vi "rethinkdb_msg_split.vi"(8 "error in (no error)":errorcluster, 11 "data in":string) -> (0 "error out":errorcluster, 2 "unterminated?":bool, 3 "messages":string[](array[string]))   [LabVIEW 2017]
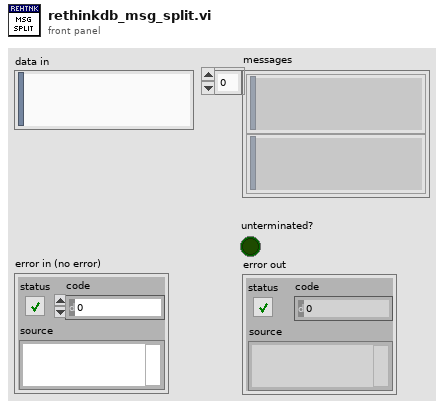
[diagram p1: front panel]
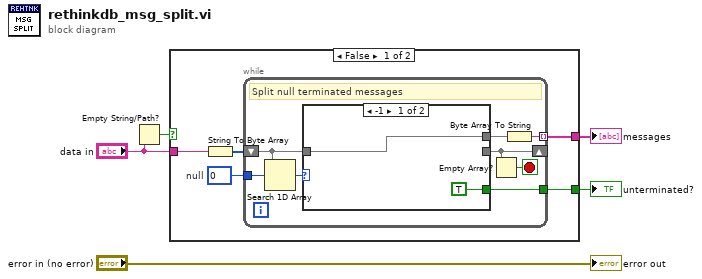
[diagram p0: block diagram]
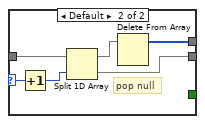
[diagram p2: hidden frame]
diagram:
  n1 = Empty String/Path?(string/path="data in") -> (empty?=w2:bool)
  n2 = case shown="False" w2 {
    tunnel: "data in" -> [w9 _]
    tunnel: [w7 _] -> w5
    tunnel: [w6 _] -> w1
    frame False {
      w10 = u8 0  # null
      n3 = String To Byte Array(string=w9) -> (unsigned byte array=w8:u8[])
      n4 = while {
        tunnel: w10 -> [w18]
        shift-right: [w13] -> _
        shift-left: w8 -> [w17]
        tunnel: [w14] -> w7 mode=indexing
        tunnel: [w11] -> w6
        stop <- w12 stop-if-true
        # "Split null terminated messages"
        n5 = Search 1D Array(1D array=w17, element=w18) -> (index of element=w16:i32)  [unwired: 1 in]
        n6 = case shown="-1" w16 {
          selector: w16 -> [_ w25]
          tunnel: w17 -> [w20 w26]
          tunnel: [_ w24] -> w13
          tunnel: [w20 w21] -> w15
          tunnel: [TRUE _] -> w11
          frame -1 {
          }
          frame Default {
            # "pop null"
            n7 = Increment(x=w25) -> (x+1=w23:i32)
            n8 = Split 1D Array(array=w26, index=w23) -> (first subarray=w22:u8[], second subarray=w24:u8[])
            n9 = Delete From Array(array=w22) -> (array with subset deleted=w21:u8[])  [unwired: 2 in, 1 out]
          }
        }
        n10 = Empty Array?(array=w13) -> (empty?=w12:bool)
        n11 = Byte Array To String(unsigned byte array=w15) -> (string=w14:string)
      }
    }
    frame True {
    }
  }
  "unterminated?" <- w1
  "messages" <- w5
  "error out" <- "error in (no error)"
